vi "TCP PXI DAQ Close Connection.vi"(8 "error in (no error)":errorcluster, 11 "connection ID":refnum<k5>) -> (0 "error out":errorcluster)   [LabVIEW 2015]
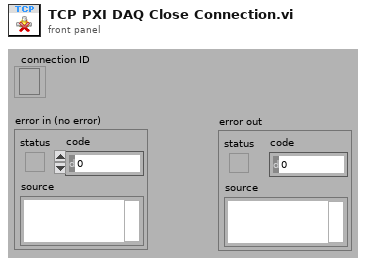
[diagram p1: front panel]
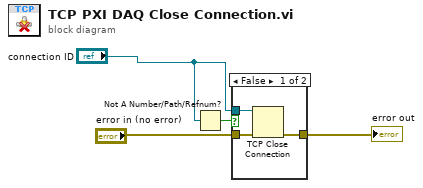
[diagram p0: block diagram]
diagram:
  n1 = Not A Number/Path/Refnum?(number/path/refnum="connection ID") -> (NaN/Path/Refnum?=w3:bool)
  n2 = case shown="False" w3 {
    tunnel: [w7 w8] -> w2
    tunnel: "error in (no error)" -> [w6 w8]
    tunnel: "connection ID" -> [w5 _]
    frame False {
      n3 = TCP Close Connection(connection ID=w5, error in (no error)=w6) -> (error out=w7:errorcluster)  [unwired: 1 in, 1 out]
    }
    frame True {
    }
  }
  "error out" <- w2
